vi "Simlated vehicle.vi"(2 "Steering angle":dbl format="%#_13g", 3 "Speed":dbl format="%#_13g") -> (0 "Steering angle sensor":dbl format="%#_13g", 1 "Speed sensor":dbl format="%#_13g")   [LabVIEW 2022 SP3]
uses:
  <vilib>/Analysis/3filter.llb/Filter Passband Type.ctl
  <vilib>/ptbypt/NI_PtbyPt.lvlib
  <vilib>/Analysis/NI_AALBase.lvlib
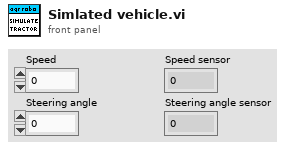
[diagram p1: front panel]
types:
  T1 = typedef "NI_AALBase.lvlib/Filter Passband Type.ctl" = enum32{"Lowpass", "Highpass", "Bandpass", "Bandstop"}
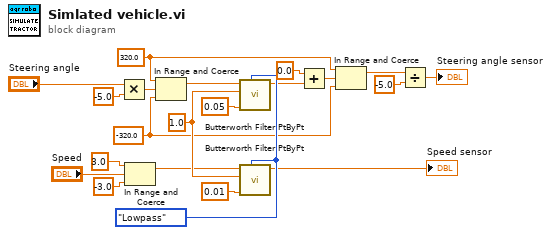
[diagram p0: block diagram]
diagram:
  w1 = -320.0 ("lower limit")
  w2 = 320.0 ("upper limit")
  w15 = Filter_Passband_Type."Lowpass" ("filter type")
  w17 = 1.0 ("sampling freq: fs")
  n1 = Multiply(x="Steering angle", y=-5.0) -> (x*y=w6:dbl)
  n2 = In Range and Coerce(upper limit=3.0, x="Speed", lower limit=-3.0) -> (coerced(x)=w13:dbl)  [unwired: 1 out]
  n3 = In Range and Coerce(upper limit=w2, x=w6, lower limit=w1) -> (coerced(x)=w14:dbl)  [unwired: 1 out]
  n4 = call <vilib>:"Butterworth Filter PtByPt.vi"("filter type"=w15, "low cutoff freq: fl"=0.05, "sampling freq: fs"=w17, "x"=w14) -> ("Filtered x"=w12:dbl)  [unwired: 5 in, 1 out]
  n5 = call <vilib>:"Butterworth Filter PtByPt.vi"("filter type"=w15, "low cutoff freq: fl"=0.01, "sampling freq: fs"=w17, "x"=w13) -> ("Filtered x"=→"Speed sensor":dbl)  [unwired: 5 in, 1 out]
  n6 = Add(x=0.0, y=w12) -> (x+y=w4:dbl)
  n7 = In Range and Coerce(upper limit=w2, x=w4, lower limit=w1) -> (coerced(x)=w3:dbl)  [unwired: 1 out]
  n8 = Divide(x=w3, y=-5.0 ("x")) -> (x/y=→"Steering angle sensor":dbl)
